vi "ParameterSampler.vi"(8 "error in (no error)":errorcluster caption="entrée d'erreur (pas d'erreur)", 11 "ParameterSampler":T1={"param_distributions"={"Key"=[], "Value"=[]}, "n_iter"=5, "random_state"=-1} {"random_state" min=-1}) -> (0 "error out":errorcluster caption="sortie d'erreur", 3 "Data":string[][](array[string]))   [LabVIEW 2020]
doc: "Generator on parameters sampled from given distributions.\n\nNon-deterministic iterable over random candidate combinations for hyper- parameter search. If all parameters are presented as a list, sampling without replacement is performed. If at least one parameter is given as a distribution, sampling with replacement is used. It is highly recommended to use continuous distributions for continuous parameters.\n\n\n\nParameters :\n\n- param_distributions : dict\nDictionary with parameters names (str) as keys and distributions or lists of parameters to try. Distributions must provide a rvs method for sampling (such as those from scipy.stats.distributions). If a list is given, it is sampled uniformly. If a list of dicts is given, first a dict is sampled uniformly, and then a parameter is sampled using that dict as above.\n\n- n_iter : integer\nNumber of parameter settings that are produced.\n\n- random_state : int or RandomState instance, default=None=-1\nPseudo random number generator state used for random uniform sampling from lists of possible values instead of scipy.stats distributions. Pass an int for reproducible output across multiple function calls. See Glossary.\n\nReturns :\n\n- params : dict of str to any\nYields dictionaries mapping each estimator parameter to as sampled value."
uses:
  ParameterSampler.lvclass
panel:
  out "ParameterSampler.lvclass":refnum<class "ParameterSampler.lvclass">
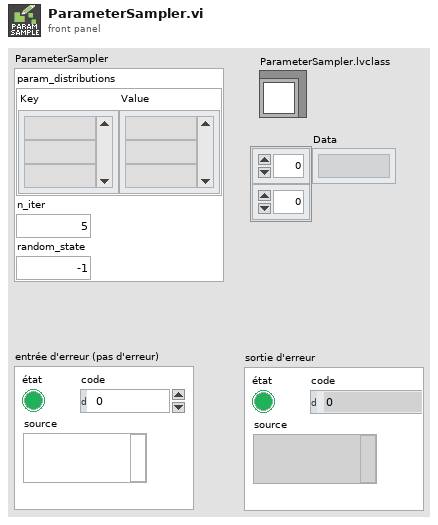
[diagram p1: front panel]
types:
  T1 = cluster{"param_distributions":cluster{"Key":string[], "Value":string[]}, "n_iter":i32, "random_state":i32}
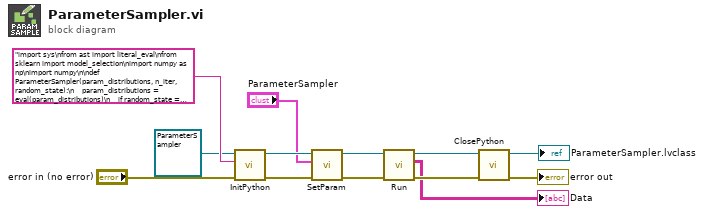
[diagram p0: block diagram]
diagram:
  n1 = call-dynamic "InitPython.vi"("error in (no error)"="error in (no error)", "Python Instruction"="import sys\nfrom ast import literal_eval\nfrom sklearn import model_selection\nimport numpy as np\nimport numpy\n\ndef ParameterSampler(param_distributions, n_iter, random_state):\n    param_distributions = eval(param_distributions)\n    if random_state == -1:\n        random_state = None\n    try:\n        ParameterSampler = model_selection.ParameterSampler(param_distributions, n_iter, random_state)\n        ParameterSampler = list(ParameterSampler)\n        return str(ParameterSampler)\n    except:\n        erreur = sys.exc_info()\n        typerr = u\"%s\" % (erreur[0])\n        typerr = typerr[typerr.find(\"'\")+1:typerr.rfind(\"'\")]\n        msgerr = u\"%s\" % (erreur[1])\n        message = str('/!\\\\ {0} : {1}'. format(typerr,msgerr))\n        return message", "Scikit-learn en entrée"=refnum<class "ParameterSampler.lvclass"> refnum ("ParameterSampler.lvclass")) -> ("error out"=w9:errorcluster, "Scikit-learn en sortie"=w8:refnum<class "ParameterSampler.lvclass">)  [unwired: 7 in]
  n2 = call-dynamic "SetParam.vi"("error in (no error)"=w9, "ParameterSampler"="ParameterSampler", "ParameterSampler.lvclass"=w8) -> ("error out"=w6:errorcluster, "ParameterSampler.lvclass"=w5:refnum<class "ParameterSampler.lvclass">)  [unwired: 7 in]
  n3 = call-dynamic "Run.vi"("error in (no error)"=w6, "ParameterSampler.lvclass"=w5) -> ("error out"=w4:errorcluster, "Data"=→"Data":string[][], "ParameterSampler.lvclass"=w3:refnum<class "ParameterSampler.lvclass">)  [unwired: 7 in]
  n4 = call-dynamic "ClosePython.vi"("error in (no error)"=w4, "Scikit-learn en entrée"=w3) -> ("error out"=→"error out":errorcluster, "Scikit-learn en sortie"=→"ParameterSampler.lvclass":refnum<class "ParameterSampler.lvclass">)  [unwired: 8 in]
